vi "SeriellReadFPGA.vi"   [LabVIEW 2017]
uses:
  <vilib>/eio/EIOMethodNode/EIOMethodNode.xnode
  <vilib>/rvi/DataTransferAndStorage/Container/XNode/niFpgaContainer.xnode
  gvboolesch.vi
  <vilib>/rvi/eio/common/nirviEmuTemplateMethod_errors.vi
  <vilib>/rvi/interface/RandomDataEmulation/nirviRandomDataFpgaReadWriteTemplate.vi
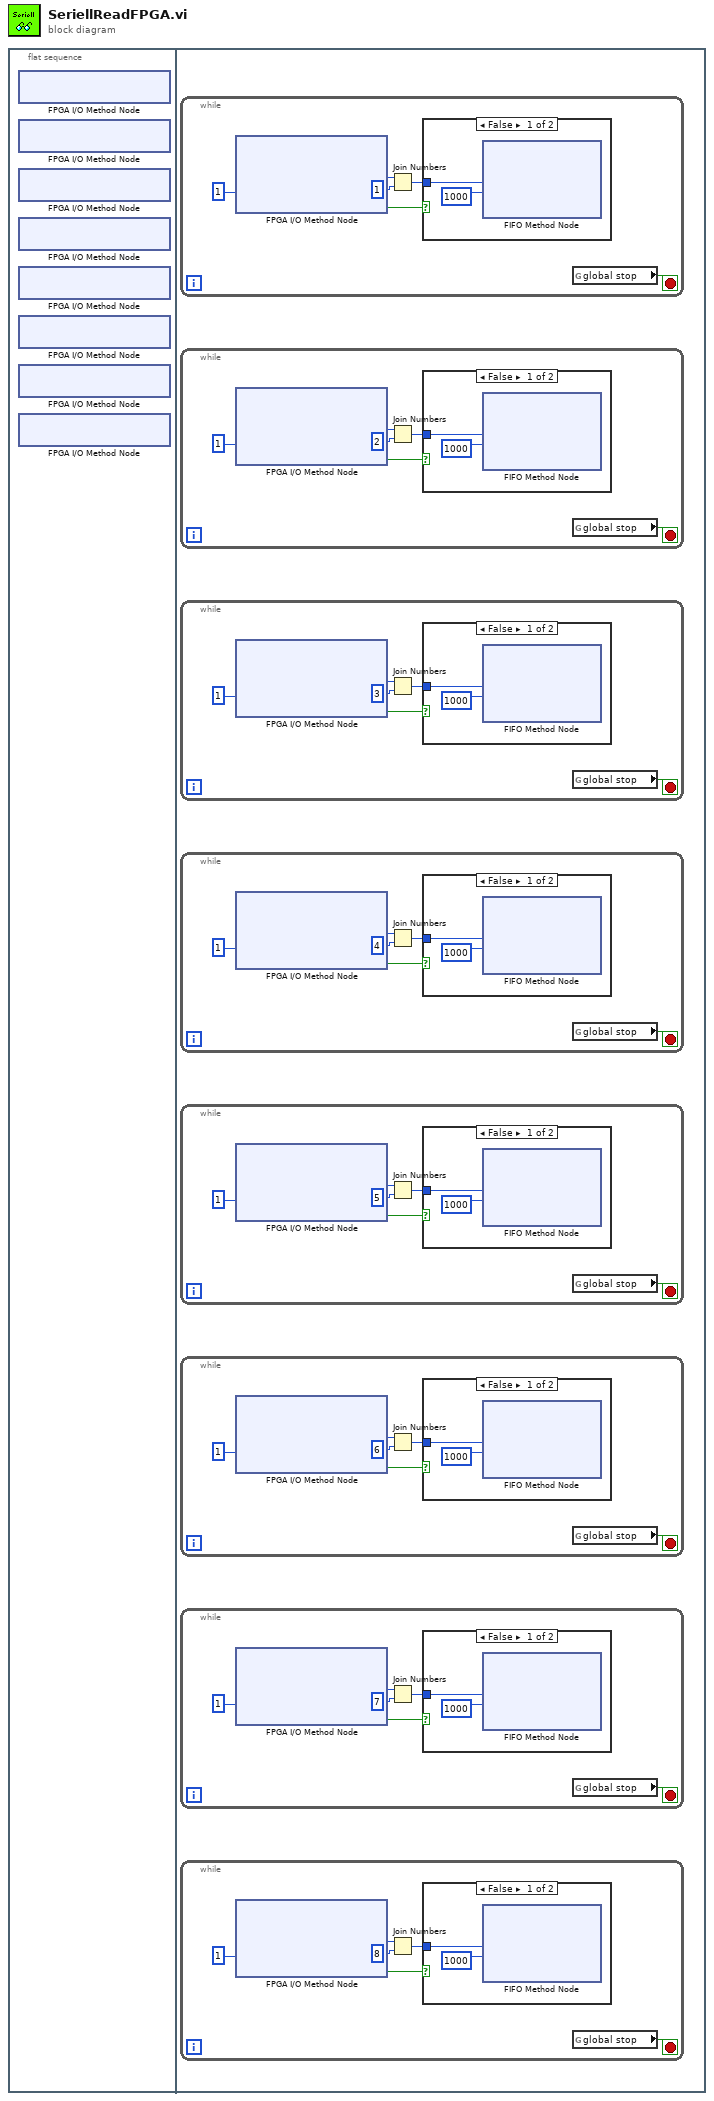
[diagram p0: block diagram]
diagram:
  n1 = flat-sequence {
    frame #0 {
      n2 = xnode "FPGA I/O Method Node"() -> ()  [unwired: 1 in, 1 out]
      n3 = xnode "FPGA I/O Method Node"() -> ()  [unwired: 1 in, 1 out]
      n4 = xnode "FPGA I/O Method Node"() -> ()  [unwired: 1 in, 1 out]
      n5 = xnode "FPGA I/O Method Node"() -> ()  [unwired: 1 in, 1 out]
      n6 = xnode "FPGA I/O Method Node"() -> ()  [unwired: 1 in, 1 out]
      n7 = xnode "FPGA I/O Method Node"() -> ()  [unwired: 1 in, 1 out]
      n8 = xnode "FPGA I/O Method Node"() -> ()  [unwired: 1 in, 1 out]
      n9 = xnode "FPGA I/O Method Node"() -> ()  [unwired: 1 in, 1 out]
    }
    frame #1 {
      n10 = while {
        stop <- w57 stop-if-true
        n11 = xnode "FPGA I/O Method Node"("Timeout (ms)"=1) -> ("Data"=w62:u8, "Timed Out"=w60:bool)  [unwired: 1 in, 1 out]
        n12 = Join Numbers(hi=w62, lo=u8 1) -> ((hi.lo)=w59:u16)
        n13 = case shown="False" w60 {
          tunnel: w59 -> [w64 _]
          frame False {
            n14 = xnode ("FIFO Method Node")("Element"=w64, "Timeout"=1000) -> ()  [unwired: 1 in, 2 out]
          }
          frame True {
          }
        }
        n15 = global read "gvboolesch.vi" "global stop"() -> (w57:bool)
      }
      n16 = while {
        stop <- w49 stop-if-true
        n17 = xnode "FPGA I/O Method Node"("Timeout (ms)"=1) -> ("Data"=w54:u8, "Timed Out"=w52:bool)  [unwired: 1 in, 1 out]
        n18 = Join Numbers(hi=w54, lo=u8 2) -> ((hi.lo)=w51:u16)
        n19 = case shown="False" w52 {
          tunnel: w51 -> [w56 _]
          frame False {
            n20 = xnode ("FIFO Method Node")("Element"=w56, "Timeout"=1000) -> ()  [unwired: 1 in, 2 out]
          }
          frame True {
          }
        }
        n21 = global read "gvboolesch.vi" "global stop"() -> (w49:bool)
      }
      n22 = while {
        stop <- w41 stop-if-true
        n23 = xnode "FPGA I/O Method Node"("Timeout (ms)"=1) -> ("Data"=w46:u8, "Timed Out"=w44:bool)  [unwired: 1 in, 1 out]
        n24 = Join Numbers(hi=w46, lo=u8 3) -> ((hi.lo)=w43:u16)
        n25 = case shown="False" w44 {
          tunnel: w43 -> [w48 _]
          frame False {
            n26 = xnode ("FIFO Method Node")("Element"=w48, "Timeout"=1000) -> ()  [unwired: 1 in, 2 out]
          }
          frame True {
          }
        }
        n27 = global read "gvboolesch.vi" "global stop"() -> (w41:bool)
      }
      n28 = while {
        stop <- w33 stop-if-true
        n29 = xnode "FPGA I/O Method Node"("Timeout (ms)"=1) -> ("Data"=w38:u8, "Timed Out"=w36:bool)  [unwired: 1 in, 1 out]
        n30 = Join Numbers(hi=w38, lo=u8 4) -> ((hi.lo)=w35:u16)
        n31 = case shown="False" w36 {
          tunnel: w35 -> [w40 _]
          frame False {
            n32 = xnode ("FIFO Method Node")("Element"=w40, "Timeout"=1000) -> ()  [unwired: 1 in, 2 out]
          }
          frame True {
          }
        }
        n33 = global read "gvboolesch.vi" "global stop"() -> (w33:bool)
      }
      n34 = while {
        stop <- w25 stop-if-true
        n35 = xnode "FPGA I/O Method Node"("Timeout (ms)"=1) -> ("Data"=w30:u8, "Timed Out"=w28:bool)  [unwired: 1 in, 1 out]
        n36 = Join Numbers(hi=w30, lo=u8 5) -> ((hi.lo)=w27:u16)
        n37 = case shown="False" w28 {
          tunnel: w27 -> [w32 _]
          frame False {
            n38 = xnode ("FIFO Method Node")("Element"=w32, "Timeout"=1000) -> ()  [unwired: 1 in, 2 out]
          }
          frame True {
          }
        }
        n39 = global read "gvboolesch.vi" "global stop"() -> (w25:bool)
      }
      n40 = while {
        stop <- w17 stop-if-true
        n41 = xnode "FPGA I/O Method Node"("Timeout (ms)"=1) -> ("Data"=w22:u8, "Timed Out"=w20:bool)  [unwired: 1 in, 1 out]
        n42 = Join Numbers(hi=w22, lo=u8 6) -> ((hi.lo)=w19:u16)
        n43 = case shown="False" w20 {
          tunnel: w19 -> [w24 _]
          frame False {
            n44 = xnode ("FIFO Method Node")("Element"=w24, "Timeout"=1000) -> ()  [unwired: 1 in, 2 out]
          }
          frame True {
          }
        }
        n45 = global read "gvboolesch.vi" "global stop"() -> (w17:bool)
      }
      n46 = while {
        stop <- w9 stop-if-true
        n47 = xnode "FPGA I/O Method Node"("Timeout (ms)"=1) -> ("Data"=w14:u8, "Timed Out"=w12:bool)  [unwired: 1 in, 1 out]
        n48 = Join Numbers(hi=w14, lo=u8 7) -> ((hi.lo)=w11:u16)
        n49 = case shown="False" w12 {
          tunnel: w11 -> [w16 _]
          frame False {
            n50 = xnode ("FIFO Method Node")("Element"=w16, "Timeout"=1000) -> ()  [unwired: 1 in, 2 out]
          }
          frame True {
          }
        }
        n51 = global read "gvboolesch.vi" "global stop"() -> (w9:bool)
      }
      n52 = while {
        stop <- w1 stop-if-true
        n53 = xnode "FPGA I/O Method Node"("Timeout (ms)"=1) -> ("Data"=w6:u8, "Timed Out"=w4:bool)  [unwired: 1 in, 1 out]
        n54 = Join Numbers(hi=w6, lo=u8 8) -> ((hi.lo)=w3:u16)
        n55 = case shown="False" w4 {
          tunnel: w3 -> [w8 _]
          frame False {
            n56 = xnode ("FIFO Method Node")("Element"=w8, "Timeout"=1000) -> ()  [unwired: 1 in, 2 out]
          }
          frame True {
          }
        }
        n57 = global read "gvboolesch.vi" "global stop"() -> (w1:bool)
      }
    }
  }
